vi "Intake Problem Fix.vi"(1 "Intake Info Modified":T1, 2 "Intake Info Original":T1) -> (0 "Intake Info Fixed":T1)   [LabVIEW 2013]
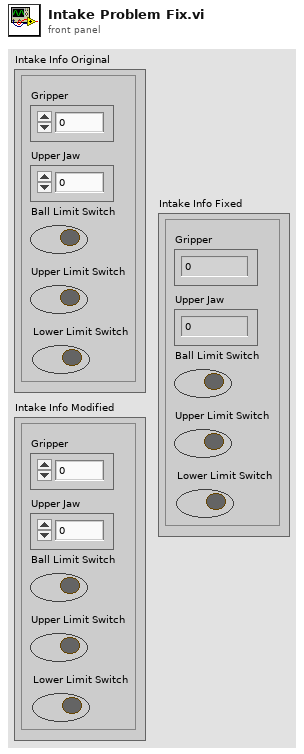
[diagram p1: front panel]
types:
  T1 = cluster{"Gripper":dbl, "Upper Jaw":dbl, "Ball Limit Switch":bool, "Upper Limit Switch":bool, "Lower Limit Switch ":bool}
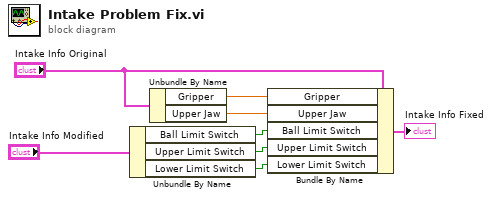
[diagram p0: block diagram]
diagram:
  n1 = Unbundle By Name("Intake Info Modified") -> ("Ball Limit Switch"=w3:bool, "Upper Limit Switch"=w2:bool, "Lower Limit Switch"=w1:bool)
  n2 = Unbundle By Name("Intake Info Original") -> ("Gripper"=w5:dbl, "Upper Jaw"=w4:dbl)
  n3 = Bundle By Name(cluster="Intake Info Original", "Gripper"=w5, "Upper Jaw"=w4, "Ball Limit Switch"=w3, "Upper Limit Switch"=w2, "Lower Limit Switch"=w1) -> (→"Intake Info Fixed":T1)
